vi "OpenNetworkGraph.vi"(8 "error in (no error)":errorcluster, 10 "ServerAddress":string, 11 "TAGS to show":string[](array[string])) -> (0 "Error out":errorcluster)   [LabVIEW 2020]
doc: "Open a New Networked Gviewer graph\n\nAndre Koelewijn, 26 June 2023\nThis vi will ask the Gserver service to open a graphic viewer to a networked Sgraph server\n(as an example, normally it is to be opened as stand-alone to a remote server)\nIf the input TAG list is used then these TAGs will show in the new graph to open.\nIf the TAG list is not wired or left empty, then a default new graph display is shown."
uses:
  Gserver/controls/Typedef_Gviewer-Query.ctl
  Gserver/controls/Typedef_QueryType.ctl
  controls/NewNetowrkGraph.ctl
  Gserver/Gserver.lvclass
  Builds/Sgraph_lib_V1.lvlib
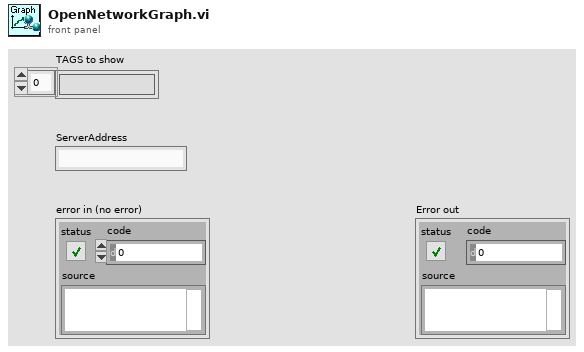
[diagram p1: front panel]
types:
  T1 = typedef "Sgraph_lib_V1.lvlib/NewNetowrkGraph.ctl" = cluster{"TAGS to show":string[], "ServerAddress":string}
  T2 = typedef "Sgraph_lib_V1.lvlib/Gserver.lvclass/Typedef_QueryType.ctl" = enum16{"Subscribe", "SubscribeNetw", "DataRequest", "RequestAllTags", "RequestIniPath", "FAMMstarted", "SetClientOptions", "GviewerUpdate", "OpenNewGraph", "CloseClient", "CloseAllClients", "Close Gserver", "OpenMemoryMap", "MeMapDataRequest", "MeMapDataResponse", "OpenDBeditor", "CheckDBeditorRunning", "StoppedDBeditor", "SaveDB_TAGpropRecord", "ConfirmDB_TAGpropSave", "GetXconstraints", "OpenNewNetworkGraph"}
  T3 = typedef "Sgraph_lib_V1.lvlib/Gserver.lvclass/Typedef_Gviewer-Query.ctl" = cluster{"Query_type":T2, "data":variant, "Source":string, "Time Stamp":timestamp}
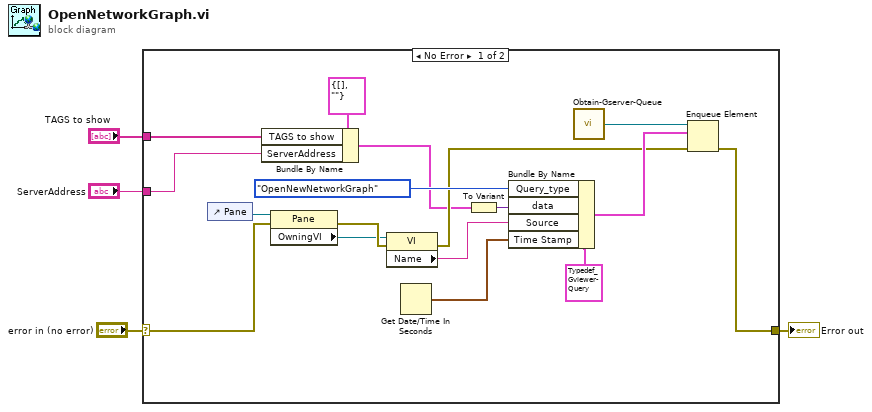
[diagram p0: block diagram]
diagram:
  n1 = case shown="No Error" "error in (no error)" {
    selector: "error in (no error)" -> [w15 w22]
    tunnel: [w12 w22] -> w3
    tunnel: "TAGS to show" -> [w7 _]
    tunnel: "ServerAddress" -> [w5 _]
    frame No Error {
      n2 = control-ref of="Pane"() -> (w17:refnum<vi>)
      n3 = Bundle By Name(cluster=T1 {"TAGS to show"=[], "ServerAddress"=""} ("Data"), "TAGS to show"=w7, "ServerAddress"=w5) -> (w6:T1)
      n4 = property class="Pane"(reference=w17, error in=w15) -> (error out=w14:errorcluster, "OwningVI"=w9:refnum<vi>)  [unwired: 1 out]
      n5 = property class="VI"(reference=w9, error in=w14) -> (error out=w13:errorcluster, "Name"=w16:string)  [unwired: 1 out]
      n6 = Get Date/Time In Seconds() -> (seconds since 1Jan1904=w11:timestamp)
      n7 = To Variant(anything=w6) -> (Variant=w10:variant)
      n8 = Bundle By Name(cluster=T3 {"Query_type"=enum."Subscribe", "data"=variant, "Source"="", "Time Stamp"=timestamp(0 s since 1904-01-01)} ("element"), "Query_type"=Typedef_QueryType."OpenNewNetworkGraph", "data"=w10, "Source"=w16, "Time Stamp"=w11) -> (w18:T3)
      n9 = call "Obtain-Gserver-Queue.vi"() -> ("Gserver Queue"=w21:refnum<queue>)  [unwired: 7 in]
      n10 = Enqueue Element(queue=w21, element=w18, error in (no error)=w13) -> (error out=w12:errorcluster)  [unwired: 1 in, 2 out]
    }
    frame Error {
    }
  }
  "Error out" <- w3
